vi "Configure Strobe.vi"(8 "error in (no error)":errorcluster, 10 "Enable Strobe (Disabled)":bool, 11 "VISA resource name":refnum<visa-resource-name>) -> (0 "error out":errorcluster, 3 "VISA resource name out":refnum<visa-resource-name>)   [LabVIEW 2024, in "Ocean Optics 2000 4000.lvlib"]
doc: "Configures the strobe to either on or off. This VI sets the Lamp Enable line (J2 pin 4)."
uses:
  Ocean Optics 2000 4000.lvlib
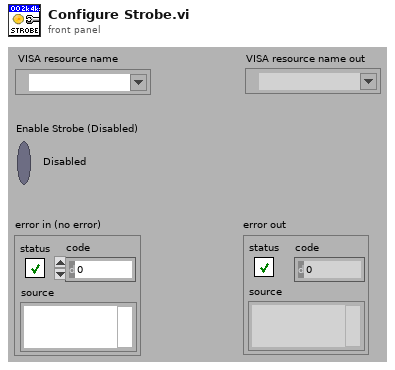
[diagram p1: front panel]
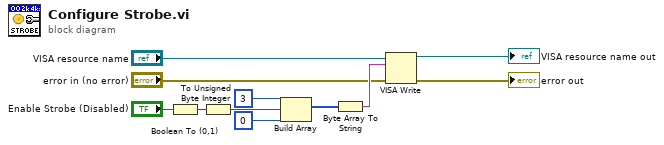
[diagram p0: block diagram]
diagram:
  n1 = Boolean To (0,1)(Boolean="Enable Strobe (Disabled)") -> (0, 1=w2:i16)
  n2 = To Unsigned Byte Integer(number=w2) -> (unsigned 8bit integer=w1:u8)
  n3 = Build Array(u8 3, w1, u8 0) -> (w10:u8[])
  n4 = Byte Array To String(unsigned byte array=w10) -> (string=w9:string)
  n5 = VISA Write(VISA resource name="VISA resource name", write buffer=w9, error in (no error)="error in (no error)") -> (VISA resource name out=→"VISA resource name out":refnum<visa-resource-name>, error out=→"error out":errorcluster)  [unwired: 1 out]
